vi "configure.vi"(8 "error in (no error)":errorcluster, 11 "YK090817SutterMP285Stage in":refnum<class "YK090817SutterMP285Stage.lvclass">=refnum) -> (0 "error out":errorcluster, 3 "YK090817SutterMP285Stage out":refnum<class "YK090817SutterMP285Stage.lvclass">)   [LabVIEW 2010, in "YK090817SutterMP285Stage.lvclass"]
doc: "The dynamic dispatch version of this VI loads and displays the configuration file associated with the plug-in object. The user modify and save the configuration data."
uses:
  YK090817SutterMP285Stage.lvclass
panel:
  in  "cancel button":bool
  in  "save button":bool
  in  "LoRes Speed (fast)":dbl=750.0
  in  "HiRes Speed (slow)":dbl=100.0
  in  "serial port #":i8
  # "Configure YK090817SutterMP285Stage"
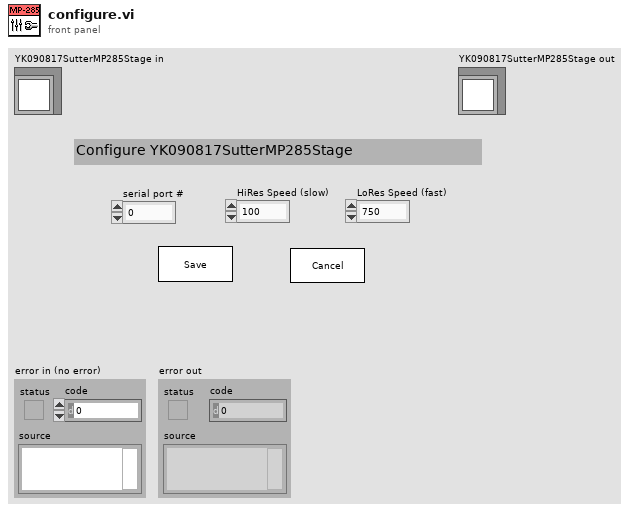
[diagram p1: front panel]
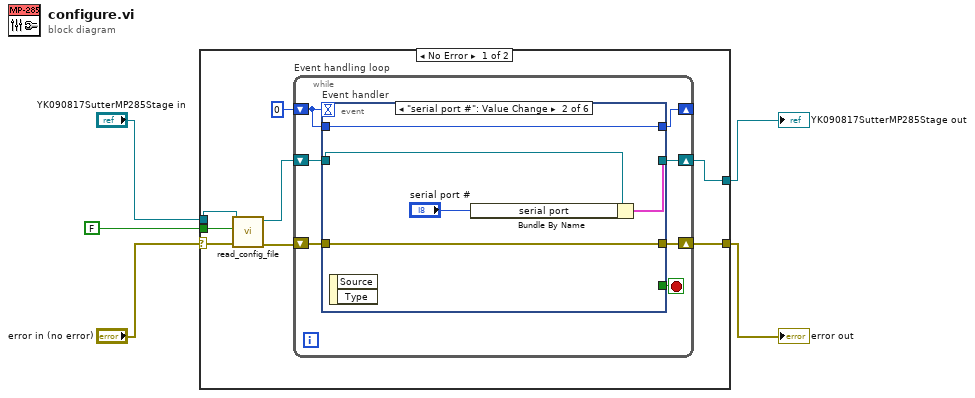
[diagram p0: block diagram]
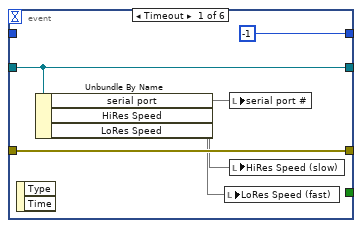
[diagram p2: hidden frame]
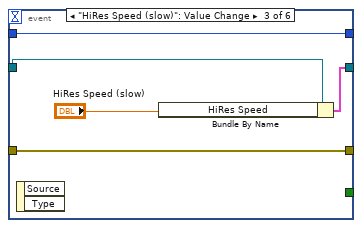
[diagram p3: hidden frame]
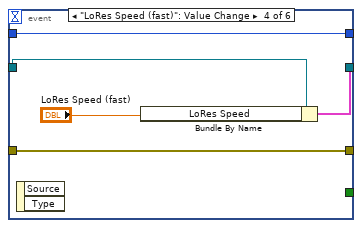
[diagram p4: hidden frame]
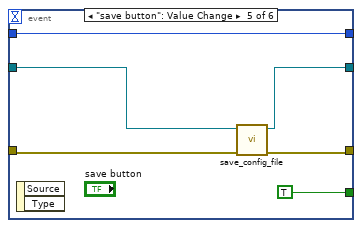
[diagram p5: hidden frame]
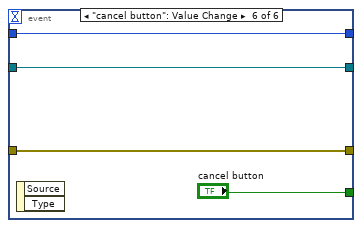
[diagram p6: hidden frame]
diagram:
  n1 = case shown="No Error" "error in (no error)" {
    selector: "error in (no error)" -> [w9 w53]
    tunnel: [w13 w53] -> w1
    tunnel: "YK090817SutterMP285Stage in" -> [w8 w52]
    tunnel: [w12 w52] -> w3
    tunnel: FALSE ("force load?") -> [w7 _]
    frame No Error {
      n2 = call-dynamic "read_config_file.vi"("error in (no error)"=w9, "force load?"=w7, "YK090817SutterMP285Stage in"=w8) -> ("error out"=w10:errorcluster, "YK090817SutterMP285Stage out"=w6:refnum<class "YK090817SutterMP285Stage.lvclass">)  [unwired: 7 out]
      n3 = while "Event handling loop" {
        shift-right: [w19] -> w13
        shift-left: w10 -> [w20]
        shift-right: [w18] -> w12
        shift-left: w6 -> [w14]
        shift-right: [w16] -> _
        shift-left: 0 -> [w17]
        stop <- w15 stop-if-true
        n4 = event "Event handler" shown="[1] \"serial port #\": Value Change" {
          selector: _ -> [_ _ _ _ _ _]
          dyn-events: _ -> [_ _ _ _ _ _]
          timeout: w17 -> [_ _ _ _ _ _]
          tunnel: w20 -> [w26 w31 w36 w41 w45 w51]
          tunnel: [w26 w31 w36 w41 w44 w51] -> w19
          tunnel: [w24 w28 w33 w38 w43 w48] -> w18
          tunnel: [-1 w30 w35 w40 w47 w50] -> w16
          tunnel: w17 -> [_ w30 w35 w40 w47 w50]
          tunnel: [_ _ _ _ TRUE "cancel button"] -> w15
          tunnel: w14 -> [w24 w29 w34 w39 w42 w48]
          event Timeout {
            n5 = event-data() -> ()  [unwired: 3 out]
            n6 = Unbundle By Name(w24) -> ("serial port"=w23, "HiRes Speed"=w22, "LoRes Speed"=w21)
            n7 = local write "LoRes Speed (fast)"(w21) -> ()
            n8 = local write "serial port #"(w23) -> ()
            n9 = local write "HiRes Speed (slow)"(w22) -> ()
          }
          event "serial port #": Value Change {
            n10 = event-data() -> ()  [unwired: 3 out]
            n11 = Bundle By Name(cluster=w29, "serial port"="serial port #") -> (w28:cluster{})
          }
          event "HiRes Speed (slow)": Value Change {
            n12 = event-data() -> ()  [unwired: 3 out]
            n13 = Bundle By Name(cluster=w34, "HiRes Speed"="HiRes Speed (slow)") -> (w33:cluster{})
          }
          event "LoRes Speed (fast)": Value Change {
            n14 = event-data() -> ()  [unwired: 3 out]
            n15 = Bundle By Name(cluster=w39, "LoRes Speed"="LoRes Speed (fast)") -> (w38:cluster{})
          }
          event "save button": Value Change {
            n16 = event-data() -> ()  [unwired: 3 out]
            n17 = call-dynamic "save_config_file.vi"("error in (no error)"=w45, "YK090817SutterMP285Stage in"=w42) -> ("error out"=w44:errorcluster, "YK090817SutterMP285Stage out"=w43:refnum<class "YK090817SutterMP285Stage.lvclass">)  [unwired: 1 in, 7 out]
          }
          event "cancel button": Value Change {
            n18 = event-data() -> ()  [unwired: 3 out]
          }
        }
      }
    }
    frame Error {
    }
  }
  "error out" <- w1
  "YK090817SutterMP285Stage out" <- w3
